vi "Update exp group.vi"(8 "error in (no error)":errorcluster, 9 "Group #":i32=-1, 10 "Experiments_group.lvclass out":refnum<class "Experiments_group.lvclass">, 11 "Control-Client in":refnum<class "Control-Client.lvclass">) -> (0 "error out":errorcluster, 3 "Control-Client out":refnum<class "Control-Client.lvclass">)   [LabVIEW 2020, in "Control-Client.lvclass"]
uses:
  Control-Client.lvclass
  Experiments/Experiments_group.lvclass
  Control-Client.lvclass/Control-Client.ctl
  Experiments/Experiments_group.lvclass/Experiments_group.ctl
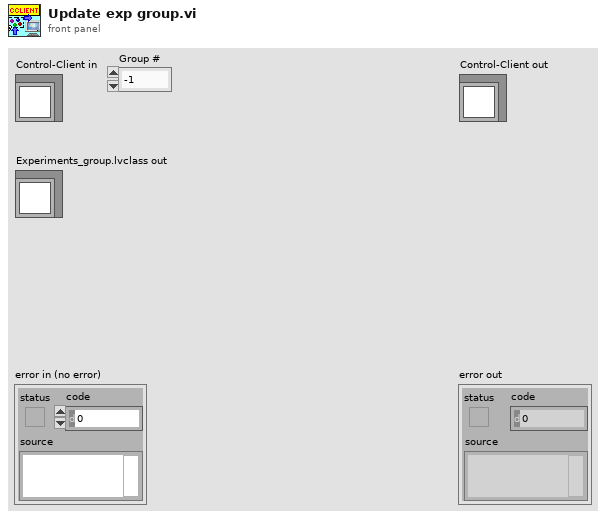
[diagram p1: front panel]
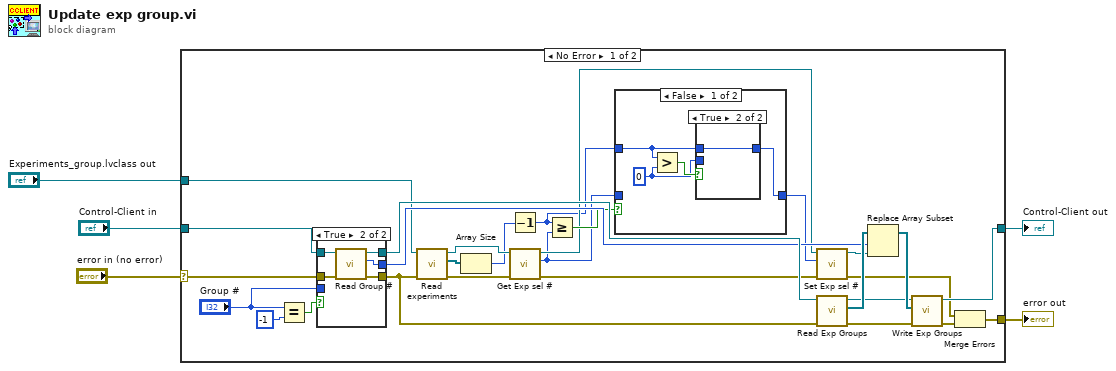
[diagram p0: block diagram]
diagram:
  n1 = case shown="No Error" "error in (no error)" {
    selector: "error in (no error)" -> [w32 w50]
    tunnel: [w7 w50] -> w4
    tunnel: [w25 w49] -> w2
    tunnel: "Control-Client in" -> [w33 w49]
    tunnel: "Experiments_group.lvclass out" -> [w6 _]
    frame No Error {
      n2 = Equal?(x="Group #", y=-1) -> (x = y?=w23:bool)
      n3 = case shown="True" w23 {
        tunnel: w33 -> [w42 w48]
        tunnel: w32 -> [w41 w47]
        tunnel: [w42 w46] -> w31
        tunnel: [w41 w45] -> w17
        tunnel: [w43 w44] -> w29
        tunnel: "Group #" -> [w43 _]
        frame False {
        }
        frame True {
          n4 = call "Read Group #.vi"("error in (no error)"=w47, "Control-Client in"=w48) -> ("error out"=w45:errorcluster, "Group #"=w44:i32, "Control-Client out"=w46:refnum<class "Control-Client.lvclass">)  [unwired: 7 in]
        }
      }
      n5 = call "Read experiments.vi"("error in (no error)"=w17, "Experiments_group.lvclass in"=w6) -> ("error out"=w18:errorcluster, "Experiments"=w20:refnum<class "Experiment.lvclass">[], "Experiments_group.lvclass out"=w21:refnum<class "Experiments_group.lvclass">)  [unwired: 6 in]
      n6 = Array Size(array=w20) -> (size(s)=w19:i32)
      n7 = Decrement(x=w19) -> (x-1=w11:i32)
      n8 = call "Get Exp sel #.vi"("error in (no error)"=w18, "Experiments_group in"=w21) -> ("error out"=w10:errorcluster, "Exp sel #"=w13:i32, "Experiments_group out"=w15:refnum<class "Experiments_group.lvclass">)  [unwired: 7 in]
      n9 = Greater Or Equal?(x=w11, y=w13) -> (x >= y?=w16:bool)
      n10 = case shown="False" w16 {
        tunnel: w13 -> [_ w40]
        tunnel: [w36 w40] -> w12
        tunnel: w11 -> [w34 _]
        frame False {
          w35 = 0 ("y")
          n11 = Greater?(x=w34, y=w35) -> (0:w37:bool)
          n12 = case shown="True" w37 {
            tunnel: [w38 w39] -> w36
            tunnel: w35 -> [w38 _]
            tunnel: w34 -> [_ w39]
            frame False {
            }
            frame True {
            }
          }
        }
        frame True {
        }
      }
      n13 = call "Set Exp sel #.vi"("error in (no error)"=w10, "Exp sel #"=w12, "Experiments_group in"=w15) -> ("error out"=w8:errorcluster, "Experiments_group out"=w14:refnum<class "Experiments_group.lvclass">)  [unwired: 7 in]
      n14 = call "Read Exp Groups.vi"("error in (no error)"=w17, "Control-Client in"=w31) -> ("error out"=w26:errorcluster, "Exp Groups"=w30:refnum<class "Experiments_group.lvclass">[], "Control-Client out"=w27:refnum<class "Control-Client.lvclass">)  [unwired: 7 in]
      n15 = Replace Array Subset(array=w30, new element=w14, index=w29) -> (w28:refnum<class "Experiments_group.lvclass">[])
      n16 = call "Write Exp Groups.vi"("error in (no error)"=w26, "Exp Groups"=w28, "Control-Client in"=w27) -> ("error out"=w9:errorcluster, "Control-Client out"=w25:refnum<class "Control-Client.lvclass">)  [unwired: 7 in]
      n17 = Merge Errors(w8, w9) -> (w7:errorcluster)
    }
    frame Error {
    }
  }
  "error out" <- w4
  "Control-Client out" <- w2
